vi "Pass If Approved.vi"(8 "error in":errorcluster, 11 "Test Data":string) -> (0 "error out":errorcluster, 2 "Failure Message":string, 3 "Passed?":bool)   [LabVIEW 2020, in "Approval Tests.lvlib"]
doc: "Performs an approval test.\n\nThe first call, the test passes and the test data is written to the approved file.\n\nOn subsequent runs the test data is compared to the contents of the approved file.\nIf it is a match, the test passes.\nIf it is not a match, the test fails and the test data is written to the actual file.\n\nAt the point the user can diff the approved and actual files and determine if they approve of the changes or not. If they approve, they replace the old approved file with the actual file. \n\nNOTE: You should keep the approved files in Source Code Control. You should ignore *.actual in your .gitignore file - there is no need to store those."
uses:
  Approval Tests.lvlib
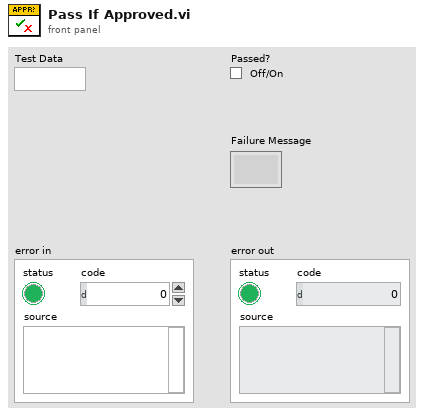
[diagram p1: front panel]
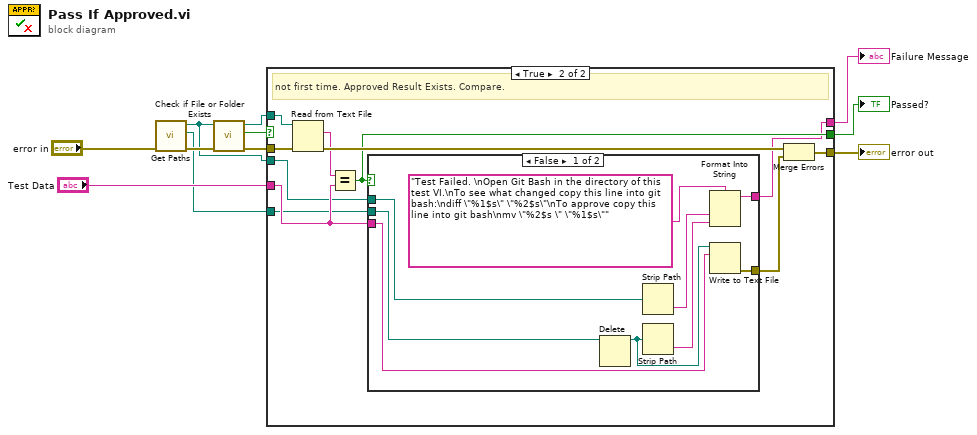
[diagram p0: block diagram]
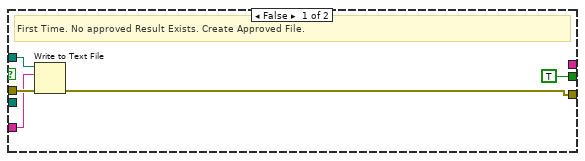
[diagram p2: hidden frame]
diagram:
  n1 = call "Get Paths.vi"("error in"="error in") -> ("error out"=w9:errorcluster, "actual path"=w3:path, "approved path"=w1:path)  [unwired: 8 in]
  n2 = call <vilib>:"Check if File or Folder Exists.vi"("error in (no error)"=w9, "path"=w1) -> ("error out"=w8:errorcluster, "file or folder exists?"=w5:bool, "dup path"=w6:path)  [unwired: 7 in]
  n3 = case shown="True" w5 {
    tunnel: "Test Data" -> [w14 w20]
    tunnel: [w16 w25] -> w11
    tunnel: w8 -> [w15 w27]
    tunnel: w6 -> [w13 w23]
    tunnel: [TRUE ("Passed?") w21] -> w4
    tunnel: w3 -> [_ w19]
    tunnel: [_ w18] -> w2
    tunnel: w1 -> [_ w17]
    frame False {
      # "First Time. No approved Result Exists. Create Approved File."
      n4 = Write to Text File(file (use dialog)=w13, text=w14, error in=w15) -> (error out=w16:errorcluster)  [unwired: 1 in, 2 out]
    }
    frame True {
      # "not first time. Approved Result Exists. Compare."
      n5 = Read from Text File(file (use dialog)=w23, error in=w27) -> (text=w22:string, error out=w26:errorcluster)  [unwired: 2 in, 2 out]
      n6 = Equal?(x=w22, y=w20) -> (x = y?=w21:bool)
      n7 = case shown="False" w21 {
        tunnel: w20 -> [w34 _]
        tunnel: w19 -> [w35 _]
        tunnel: [w36 _] -> w24
        tunnel: [w33 _] -> w18
        tunnel: w17 -> [w29 _]
        frame False {
          n8 = Delete(path (use dialog)=w35) -> (deleted path=w28:path)  [unwired: 4 in, 2 out]
          n9 = Strip Path(path=w29) -> (name=w31:string)  [unwired: 1 out]
          n10 = Strip Path(path=w28) -> (name=w30:string)  [unwired: 1 out]
          n11 = Format Into String(format string="Test Failed. \nOpen Git Bash in the directory of this test VI.\nTo see what changed copy this line into git bash:\ndiff \"%1$s\" \"%2$s\"\nTo approve copy this line into git bash\nmv \"%2$s \" \"%1$s\"", w31, w30) -> (resulting string=w33:string)  [unwired: 2 in, 1 out]
          n12 = Write to Text File(file (use dialog)=w28, text=w34) -> (error out=w36:errorcluster)  [unwired: 2 in, 2 out]
        }
        frame True {
        }
      }
      n13 = Merge Errors(w26, w24) -> (w25:errorcluster)
    }
  }
  "error out" <- w11
  "Passed?" <- w4
  "Failure Message" <- w2
